vi "Gyro controls.vi"(10 "Reset":bool, 11 "Enum":T1) -> (3 "Angle":dbl)   [LabVIEW 2014]
uses:
  SRE Enum.ctl
  <vilib>/Rock Robotics/SystemInterfaces/AI/FPGA_AIGyroChannel.ctl
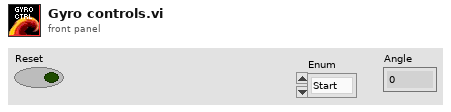
[diagram p1: front panel]
types:
  T1 = typedef "SRE Enum.ctl" = enum16{"Start", "Run", "End"}
  T2 = typedef "FPGA_AIGyroChannel.ctl" = enum8{"AI 0", "AI 1", "Invalid"}
  T3 = typedef "WPI_GyroDevRef.ctl" = cluster{"DevStatus":errorcluster, "Analog Module":T4, "Analog Channel":T5, "Offset":dbl, "Gain (VoltsPerDegree/Second)":dbl}
  T4 = typedef "FPGA_TypedefAnalogModule.ctl" = enum16{"Controller 1"}
  T5 = typedef "FPGA_AIChannel.ctl" = enum8{"AI 0", "AI 1", "AI 2", "AI 3", "AI MXP 0", "AI MXP 1", "AI MXP 2", "AI MXP 3", "Invalid"}
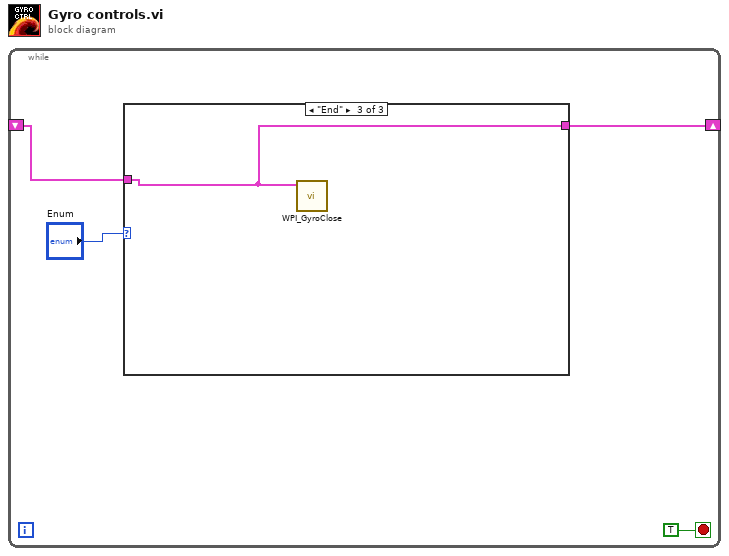
[diagram p0: block diagram]
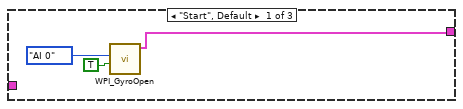
[diagram p2: hidden frame]
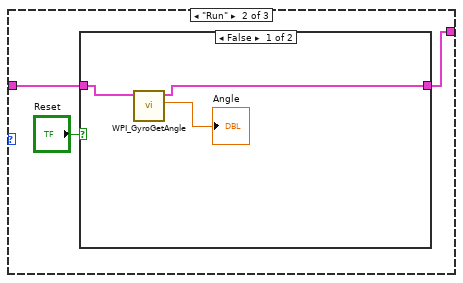
[diagram p3: hidden frame]
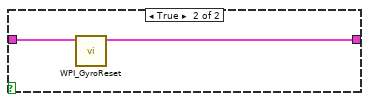
[diagram p4: hidden frame]
diagram:
  n1 = while {
    shift-right: [w3] -> _
    shift-left: _ -> [w2]
    stop <- TRUE stop-if-true
    n2 = case shown="\"End\"" "Enum" {
      tunnel: [w5 w8 w16] -> w3
      tunnel: w2 -> [_ w9 w16]
      frame "Start", Default {
        n3 = call <vilib>:"WPI_GyroOpen.vi"("Calibrate On Open"=TRUE, "Analog Channel"=FPGA_AIGyroChannel."AI 0") -> ("GyroDevRef"=w5:T3)  [unwired: 7 in, 2 out]
      }
      frame "Run" {
        n4 = case shown="False" "Reset" {
          tunnel: w9 -> [w13 w15]
          tunnel: [w12 w14] -> w8
          frame False {
            n5 = call <vilib>:"WPI_GyroGetAngle.vi"("GyroDevRef"=w13) -> ("Angle"=→"Angle":dbl, "GyroDevRef"=w12:T3)  [unwired: 7 in, 2 out]
          }
          frame True {
            n6 = call <vilib>:"WPI_GyroReset.vi"("GyroDevRef"=w15) -> ("GyroDevRef"=w14:T3)  [unwired: 9 in, 1 out]
          }
        }
      }
      frame "End" {
        n7 = call <vilib>:"WPI_GyroClose.vi"("GyroDevRef"=w16) -> ()  [unwired: 10 in, 1 out]
      }
    }
  }
